vi "fitting_padding_array.vi"(11 "array in":ext[](array[numeric])) -> (3 "Array out":ext[](array[numeric]))   [LabVIEW 2017]
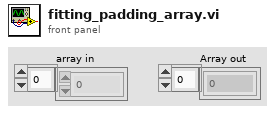
[diagram p1: front panel]
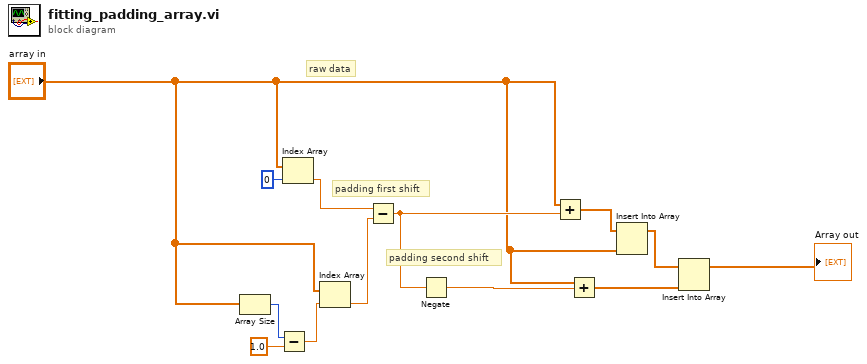
[diagram p0: block diagram]
diagram:
  # "padding second shift"
  # "padding first shift"
  # "raw data"
  n1 = Array Size(array="array in") -> (size(s)=w6:i32)
  n2 = Subtract(x=w6, y=1.0) -> (x-y=w7:dbl)
  n3 = Index Array(array="array in", index=0) -> (element=w8:ext)
  n4 = Index Array(array="array in", index=w7) -> (element=w9:ext)
  n5 = Subtract(x=w8, y=w9) -> (x-y=w2:ext)
  n6 = Negate(x=w2) -> (-x=w3:ext)
  n7 = Add(x="array in", y=w2) -> (x+y=w11:ext[])
  n8 = Add(x="array in", y=w3) -> (x+y=w12:ext[])
  n9 = Insert Into Array(array=w11, new element="array in") -> (w10:ext[])  [unwired: 1 in]
  n10 = Insert Into Array "Insert Into Array"(array=w10, new element=w12) -> (→"Array out":ext[])  [unwired: 1 in]
